vi "Single Register.vi"() -> ()   [LabVIEW 2024, in "Logging.lvlib"]
uses:
  Logging.lvlib
  Registry.lvlib
  Logger/Logger.lvclass
panel:
  out "register test":bool
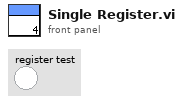
[diagram p1: front panel]
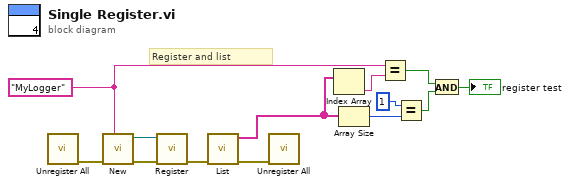
[diagram p0: block diagram]
diagram:
  w9 = "MyLogger" ("name")
  # "Register and list"
  n1 = call "Unregister All.vi"() -> ("error out"=w3:errorcluster)  [unwired: 10 in, 1 out]
  n2 = call "New.vi"("name"=w9, "error in (no error)"=w3) -> ("error out"=w5:errorcluster, "logger"=w13:refnum<class "Logger.lvclass">)  [unwired: 8 in]
  n3 = call "Register.vi"("error in (no error)"=w5, "logger in"=w13) -> ("error out"=w4:errorcluster)  [unwired: 9 in]
  n4 = call "List.vi"("error in (no error)"=w4) -> ("error out"=w2:errorcluster, "registered loggers"=w1:string[])  [unwired: 9 in]
  n5 = call "Unregister All.vi"("error in (no error)"=w2) -> ()  [unwired: 9 in, 2 out]
  n6 = Index Array(array=w1) -> (element=w10:string)  [unwired: 1 in]
  n7 = Array Size(array=w1) -> (size(s)=w12:i32)
  n8 = Equal?(x=w9, y=w10) -> (x = y?=w8:bool)
  n9 = Equal?(x=1, y=w12) -> (x = y?=w7:bool)
  n10 = And(x=w8, y=w7) -> (x .and. y?=→"register test":bool)
